vi "PathPlanner_Path_ToPathFile.vi"(9 "FileName":string="path1.path", 11 "PathPlannerPath":T7={"Reversed"=FALSE, "RotationTargets"=[], "ConstraintZones"=[], "EventMarkers"=[], "GlobalConstraints"={"MaxVelocityMps;"=0.0, "MaxAccelerationMpsSq;"=0.0, "MaxAngularVelRadPsEc;"=0.0, "MaxAngularAccRadPSecSq"=0.0, "Exists"=FALSE, "Unlimited"=FALSE, "NominalVoltageVolts"=12.0}, "GoalEndState"={"VelocityMPS"=0.0, "Rotation"={"VALUE"=0.0, "COS"=1.0, "SIN"=0.0}}, "AllPoints"=[], "Name"="", "Waypoints"=[], "PointTowardsZones"=[], "IdealStartingState"={"VelocityMPS"=0.0, "Rotation"={"VALUE"=1.0, "COS"=0.0, "SIN"=0.0}}, "IsChoreoPath"=FALSE, "PreventFlipping"=FALSE} {"IdealStartingState"."Rotation"."SIN" format="%13.4f"; "IdealStartingState"."Rotation"."COS" format="%13.4f"; "IdealStartingState"."Rotation"."VALUE" format="%13.4f"; "PointTowardsZones"."TargetPosition"."Y" format="%14.3f"; "PointTowardsZones"."TargetPosition"."X" format="%14.3f"; "PointTowardsZones"."RotationOffset"."SIN" format="%13.4f"; "PointTowardsZones"."RotationOffset"."COS" format="%13.4f"; "PointTowardsZones"."RotationOffset"."VALUE" format="%13.4f"; "Waypoints"."nextControl"."Y" format="%14.3f"; "Waypoints"."nextControl"."X" format="%14.3f"; "Waypoints"."anchor"."Y" format="%14.3f"; "Waypoints"."anchor"."X" format="%14.3f"; "Waypoints"."prevControl"."Y" format="%14.3f"; "Waypoints"."prevControl"."X" format="%14.3f"; "AllPoints"."RotationTarget"."rotation"."SIN" format="%13.4f"; "AllPoints"."RotationTarget"."rotation"."COS" format="%13.4f"; "AllPoints"."RotationTarget"."rotation"."VALUE" format="%13.4f"; "AllPoints"."Position"."Y" format="%14.3f"; "AllPoints"."Position"."X" format="%14.3f"; "GoalEndState"."Rotation"."SIN" format="%13.4f"; "GoalEndState"."Rotation"."COS" format="%13.4f"; "GoalEndState"."Rotation"."VALUE" format="%13.4f"; "RotationTargets"."rotation"."SIN" format="%13.4f"; "RotationTargets"."rotation"."COS" format="%13.4f"; "RotationTargets"."rotation"."VALUE" format="%13.4f"}) -> (0 "error out":errorcluster, 4 "Full Filename":string)   [LabVIEW 2019, in "PathPlanner24.lvlib"]
doc: "Write a path to a path file in storage. The path normally has a .PATH extension. Internally this file is formatted as JSON.\n\nInputs: \n - Path - cluster - PathPlannerPath created from the given file name\n - filename - string - The name of the path to write. Existing files will be overwritten.\n\nOutputs:\n - Error out - cluster - Error cluster\n - Full Filename - string - fully qualified file name.\n\nNotes on file naming:\n - The file name must include the extention. \".csv\" is not automatically appended to the name. \n - The file name can be a simple file or an absolute path. If a simple file name is used the default path on the RoboRIO is: \"home:\\lvuser\\natinst\\LabVIEW Data\". On a Windows PC the default path is the LabVIEW default directory. Normally this is: “%HOMEDRIVE%%HOMEPATH%\\Documents\\LabView Data\".\n - Filenames on the RoboRIO, which runs Linux, are case sensitive."
uses:
  PathPlanner24.lvlib
  TypeDef/PathPlannerPath.ctl
  TypeDef/PathPlannerRotationTarget.ctl
  <vilib>/Rock Robotics/WPI/ThirdParty/JAS_Junk/TrajLib/TypeDef/ROTATION2D.ctl
  TypeDef/PathPlannerConstraintsZone.ctl
  TypeDef/PathPlannerPathConstraints.ctl
  TypeDef/PathPlannerEventMarker.ctl
  TypeDef/PathPlannerCommandUtil.ctl
  ENum/PathPlanner_CommandUtil_Type_ENUM.ctl
  TypeDef/PathPlannerGoalEndState.ctl
  TypeDef/PathPlannerPathPoint.ctl
  <vilib>/Rock Robotics/WPI/ThirdParty/JAS_Junk/TrajLib/TypeDef/TRANSLATION2D.ctl
  TypeDef/PathPlannerWaypoint.ctl
  TypeDef/PathPlannerPointTowardsZone.ctl
  TypeDef/PathPlannerIdealStartingState.ctl
  <vilib>/Rock Robotics/WPI/ThirdParty/JAS_Junk/TrajLib/Rotation2d_GetRadians.vi
  <vilib>/Rock Robotics/WPI/ThirdParty/JAS_Junk/TrajLib/Conv_Radians_Deg.vi
  <vilib>/Rock Robotics/WPI/ThirdParty/JAS_Junk/TrajLib/Trajectory_Library.lvlib
panel:
  in  "?":T1={"name"="", "waypointRelativePos"=0.0, "command"={"type"="", "data"={"commands"=[]}}, "endWaypointRelativePos"=-1.0}
  in  "constraintZones 2":T2
  in  "waypoint":T3={"anchor"={"x"=1e+30, "y"=1e+31}, "prevControl"={"x"=1e+30, "y"=1e+31}, "nextControl"={"x"=1e+30, "y"=1e+31}, "isLocked"=FALSE}
  out "JSON string":string
  in  "constraintZones":T4
  in  "?":T5
  in  "?":T6={"version"="2025.0", "reversed"=FALSE, "globalConstraints"={"maxVelocity"=1.0, "maxAcceleration"=1.0, "maxAngularVelocity"=1.0, "maxAngularAcceleration"=1.0, "nominalVoltage"=1.0, "unlimited"=FALSE}, "goalEndState"={"velocity"=1.0, "rotation"=1.0}, "waypoints"=[], "constraintZones"=[], "rotationTargets"=[], "idealStartingState"={"velocity"=0.0, "rotation"=0.0}, "pointTowardsZones"=[], "useDefaultConstraints"=FALSE, "eventMarkers"=[]}
  in  "error in (no error)":errorcluster
  # "Constraint Zones"
  # "PointTowardsZones"
  # "Rotation Targets"
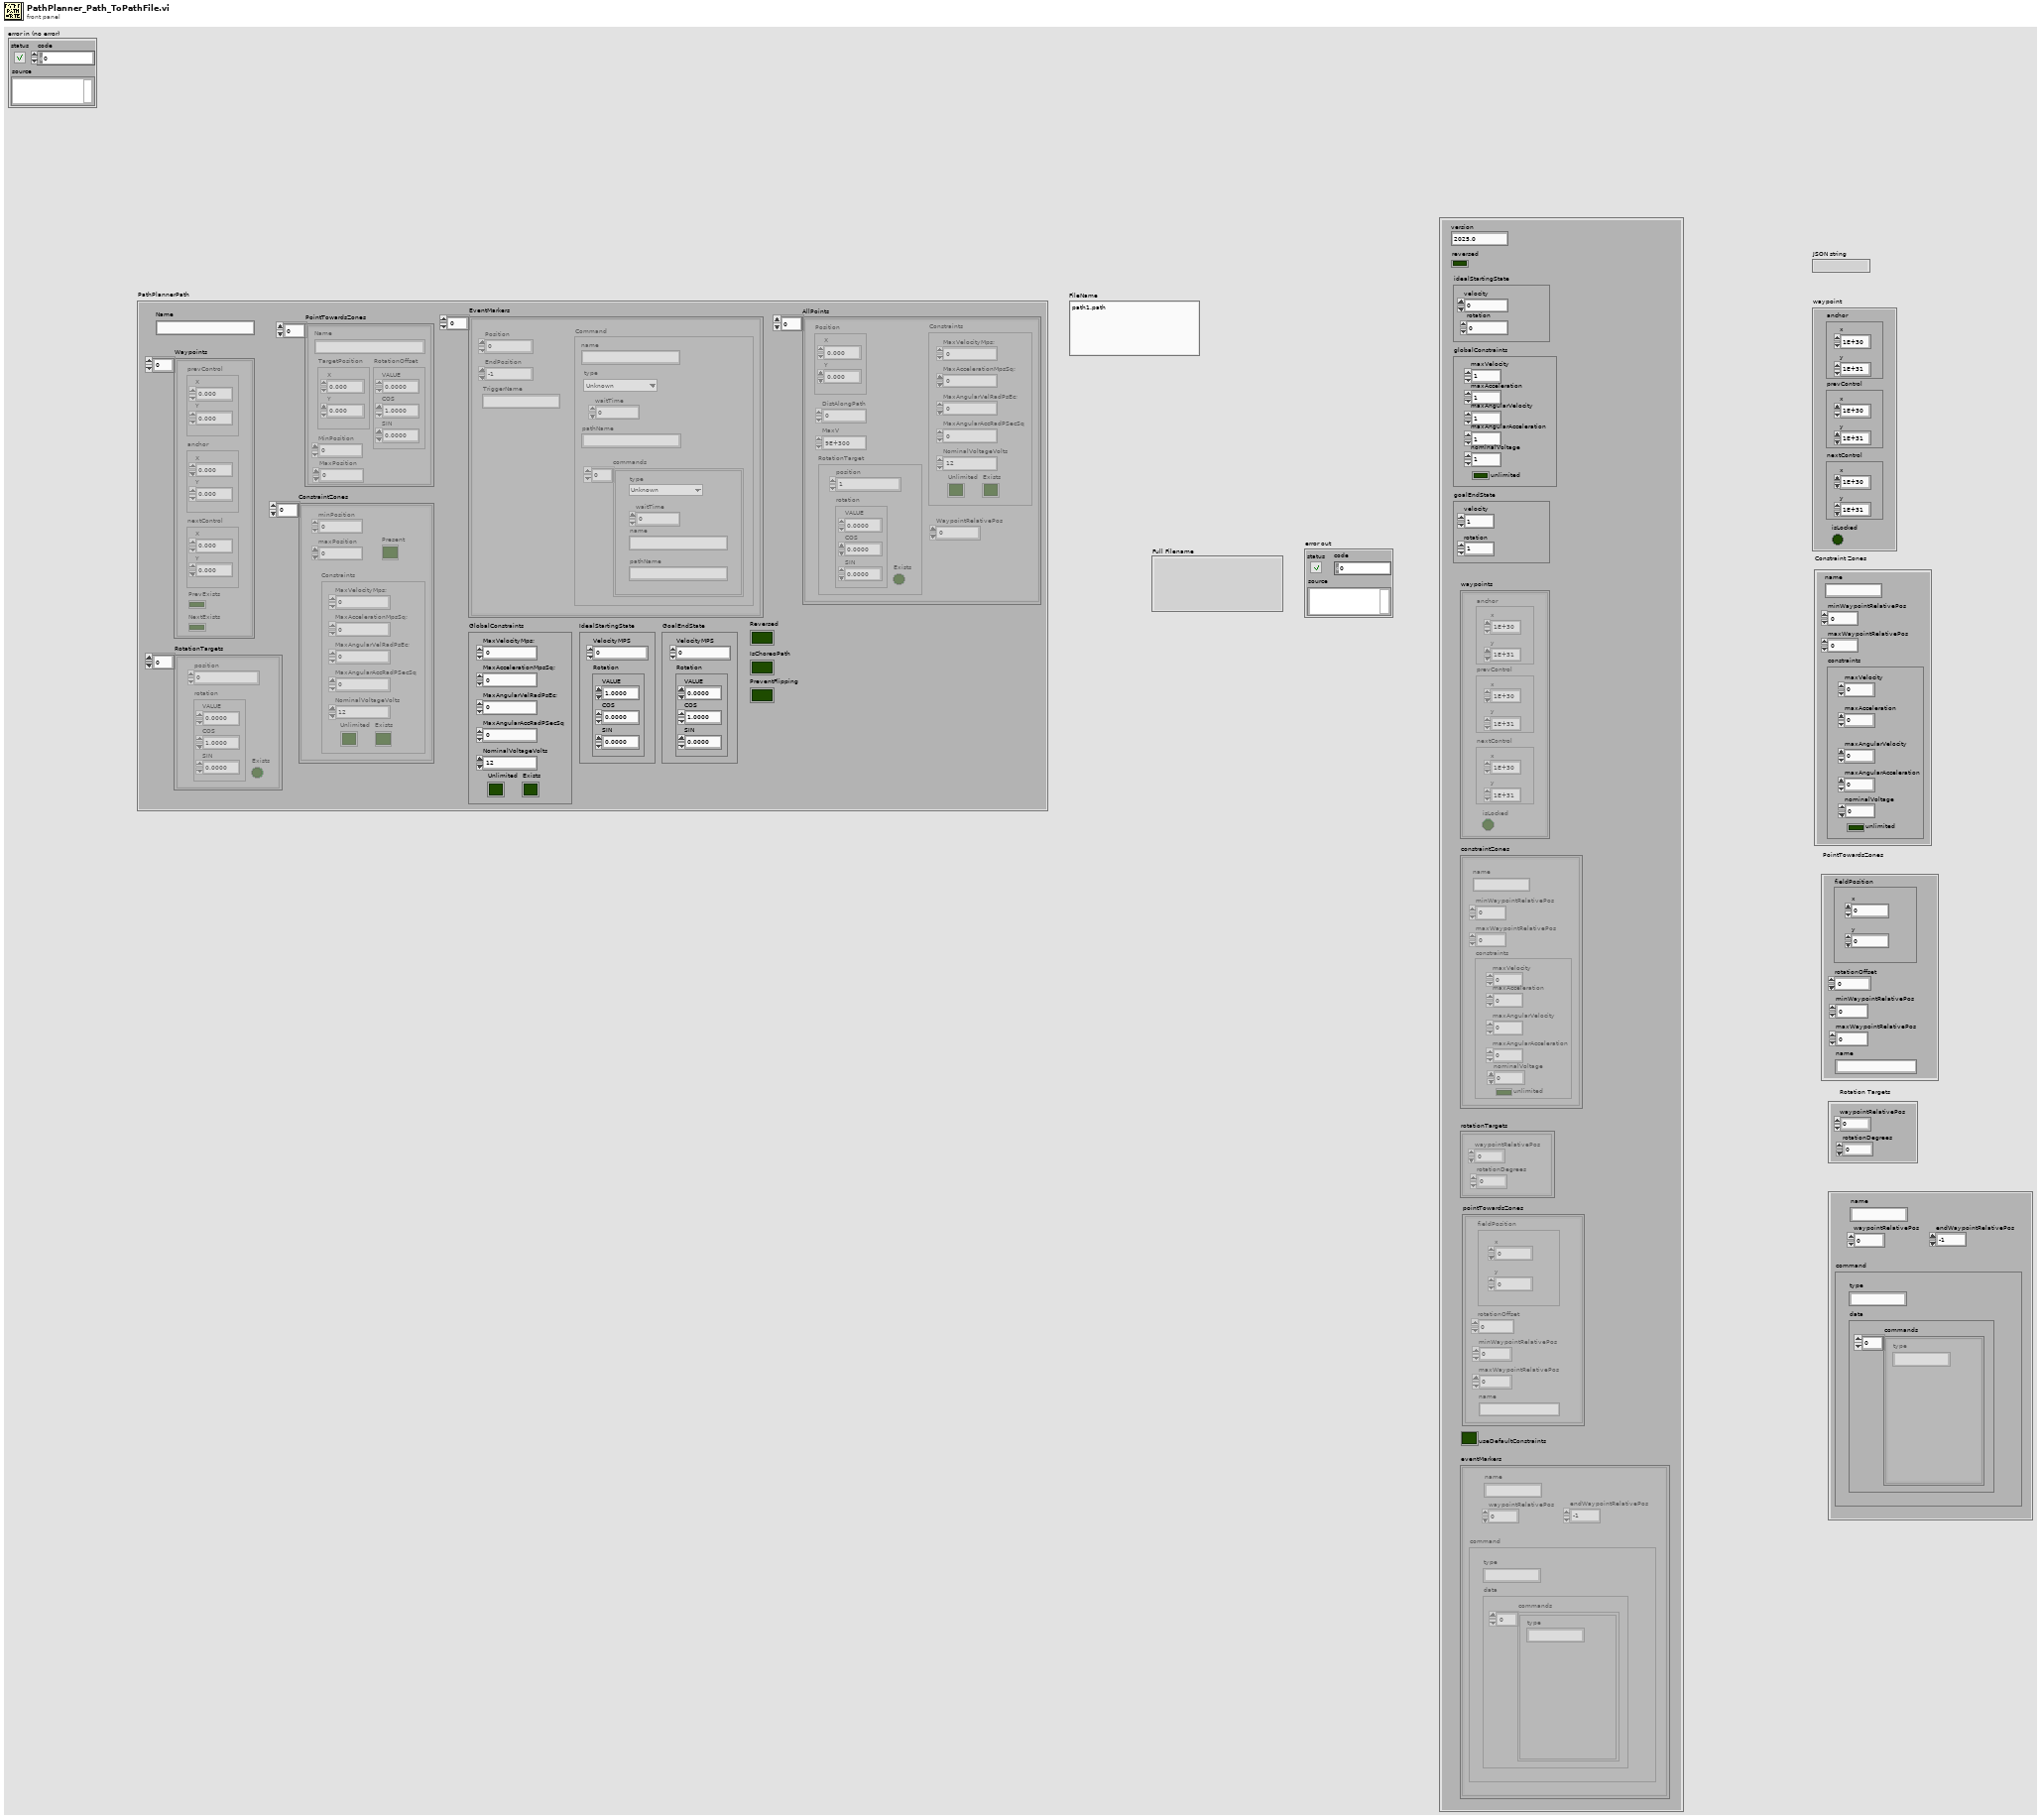
[diagram p1: front panel]
types:
  T1 = cluster{"name":string, "waypointRelativePos":dbl, "command":cluster{"type":string, "data":cluster{"commands":cluster{"type":string}[]}}, "endWaypointRelativePos":dbl}
  T2 = cluster{"fieldPosition":cluster{"x":dbl, "y":dbl}, "rotationOffset":dbl, "minWaypointRelativePos":dbl, "maxWaypointRelativePos":dbl, "name":string}
  T3 = cluster{"anchor":cluster{"x":dbl, "y":dbl}, "prevControl":cluster{"x":dbl, "y":dbl}, "nextControl":cluster{"x":dbl, "y":dbl}, "isLocked":bool}
  T4 = cluster{"name":string, "minWaypointRelativePos":dbl, "maxWaypointRelativePos":dbl, "constraints":cluster{"maxVelocity":dbl, "maxAcceleration":dbl, "maxAngularVelocity":dbl, "maxAngularAcceleration":dbl, "nominalVoltage":dbl, "unlimited":bool}}
  T5 = cluster{"waypointRelativePos":dbl, "rotationDegrees":dbl}
  T6 = cluster{"version":string, "reversed":bool, "globalConstraints":cluster{"maxVelocity":dbl, "maxAcceleration":dbl, "maxAngularVelocity":dbl, "maxAngularAcceleration":dbl, "nominalVoltage":dbl, "unlimited":bool}, "goalEndState":cluster{"velocity":dbl, "rotation":dbl}, "waypoints":cluster{"anchor":cluster{"x":dbl, "y":dbl}, "prevControl":cluster{"x":dbl, "y":dbl}, "nextControl":cluster{"x":dbl, "y":dbl}, "isLocked":bool}[], "constraintZones":cluster{"name":string, "minWaypointRelativePos":dbl, "maxWaypointRelativePos":dbl, "constraints":cluster{"maxVelocity":dbl, "maxAcceleration":dbl, "maxAngularVelocity":dbl, "maxAngularAcceleration":dbl, "nominalVoltage":dbl, "unlimited":bool}}[], "rotationTargets":cluster{"waypointRelativePos":dbl, "rotationDegrees":dbl}[], "idealStartingState":cluster{"velocity":dbl, "rotation":dbl}, "pointTowardsZones":cluster{"fieldPosition":cluster{"x":dbl, "y":dbl}, "rotationOffset":dbl, "minWaypointRelativePos":dbl, "maxWaypointRelativePos":dbl, "name":string}[], "useDefaultConstraints":bool, "eventMarkers":cluster{"name":string, "waypointRelativePos":dbl, "command":cluster{"type":string, "data":cluster{"commands":cluster{"type":string}[]}}, "endWaypointRelativePos":dbl}[]}
  T7 = typedef "PathPlanner24.lvlib/PathPlannerPath.ctl" = cluster{"Reversed":bool, "RotationTargets":T8[], "ConstraintZones":T10[], "EventMarkers":T12[], "GlobalConstraints":T11, "GoalEndState":T15, "AllPoints":T16[], "Name":string, "Waypoints":T18[], "PointTowardsZones":T19[], "IdealStartingState":T20, "IsChoreoPath":bool, "PreventFlipping":bool}
  T8 = typedef "PathPlanner24.lvlib/PathPlannerRotationTarget.ctl" = cluster{"position":dbl, "rotation":T9, "Exists":bool}
  T9 = typedef "Trajectory_Library.lvlib/ROTATION2D.ctl" = cluster{"VALUE":dbl, "COS":dbl, "SIN":dbl}
  T10 = typedef "PathPlanner24.lvlib/PathPlannerConstraintsZone.ctl" = cluster{"minPosition":dbl, "maxPosition":dbl, "Constraints":T11, "Present":bool}
  T11 = typedef "PathPlanner24.lvlib/PathPlannerPathConstraints.ctl" = cluster{"MaxVelocityMps;":dbl, "MaxAccelerationMpsSq;":dbl, "MaxAngularVelRadPsEc;":dbl, "MaxAngularAccRadPSecSq":dbl, "Exists":bool, "Unlimited":bool, "NominalVoltageVolts":dbl}
  T12 = typedef "PathPlanner24.lvlib/PathPlannerEventMarker.ctl" = cluster{"Position":dbl, "Command":T13, "TriggerName":string, "EndPosition":dbl}
  T13 = typedef "PathPlanner24.lvlib/PathPlannerCommandUtil.ctl" = cluster{"waitTime":dbl, "name":string, "pathName":string, "commands":cluster{"type":T14, "waitTime":dbl, "name":string, "pathName":string}[], "type":T14}
  T14 = typedef "PathPlanner24.lvlib/PathPlanner_CommandUtil_Type_ENUM.ctl" = enum16{"Unknown", "Wait", "Named", "Path", "Sequential", "Parallel", "Race", "Deadline", "PointTowardsZoneEnter", "PointTowardsZoneExit", "TriggerEventStart", "TriggerEventStop", "TriggerEventOneshot"}
  T15 = typedef "PathPlanner24.lvlib/PathPlannerGoalEndState.ctl" = cluster{"VelocityMPS":dbl, "Rotation":T9}
  T16 = typedef "PathPlanner24.lvlib/PathPlannerPathPoint.ctl" = cluster{"Position":T17, "DistAlongPath":dbl, "MaxV":dbl, "Constraints":T11, "RotationTarget":T8, "WaypointRelativePos":dbl}
  T17 = typedef "Trajectory_Library.lvlib/TRANSLATION2D.ctl" = cluster{"X":dbl, "Y":dbl}
  T18 = typedef "PathPlanner24.lvlib/PathPlannerWaypoint.ctl" = cluster{"prevControl":T17, "anchor":T17, "nextControl":T17, "PrevExists":bool, "NextExists":bool}
  T19 = typedef "PathPlanner24.lvlib/PathPlannerPointTowardsZone.ctl" = cluster{"RotationOffset":T9, "Name":string, "TargetPosition":T17, "MinPosition":dbl, "MaxPosition":dbl}
  T20 = typedef "PathPlanner24.lvlib/PathPlannerIdealStartingState.ctl" = cluster{"VelocityMPS":dbl, "Rotation":T9}
  T21 = cluster{"name":string, "waypointRelativePos":dbl, "command":cluster{"type":string, "data":cluster{"commands":cluster{"type":string}[]}}, "endWaypointRelativePos":dbl}[]
  T22 = cluster{"name":string, "minWaypointRelativePos":dbl, "maxWaypointRelativePos":dbl, "constraints":cluster{"maxVelocity":dbl, "maxAcceleration":dbl, "maxAngularVelocity":dbl, "maxAngularAcceleration":dbl, "nominalVoltage":dbl, "unlimited":bool}}[]
  T23 = cluster{"waypointRelativePos":dbl, "rotationDegrees":dbl}[]
  T24 = cluster{"fieldPosition":cluster{"x":dbl, "y":dbl}, "rotationOffset":dbl, "minWaypointRelativePos":dbl, "maxWaypointRelativePos":dbl, "name":string}[]
  T25 = cluster{"anchor":cluster{"x":dbl, "y":dbl}, "prevControl":cluster{"x":dbl, "y":dbl}, "nextControl":cluster{"x":dbl, "y":dbl}, "isLocked":bool}[]
  T26 = enum16{"open", "replace", "create", "open or create", "replace or create", "replace or create with confirmation"}
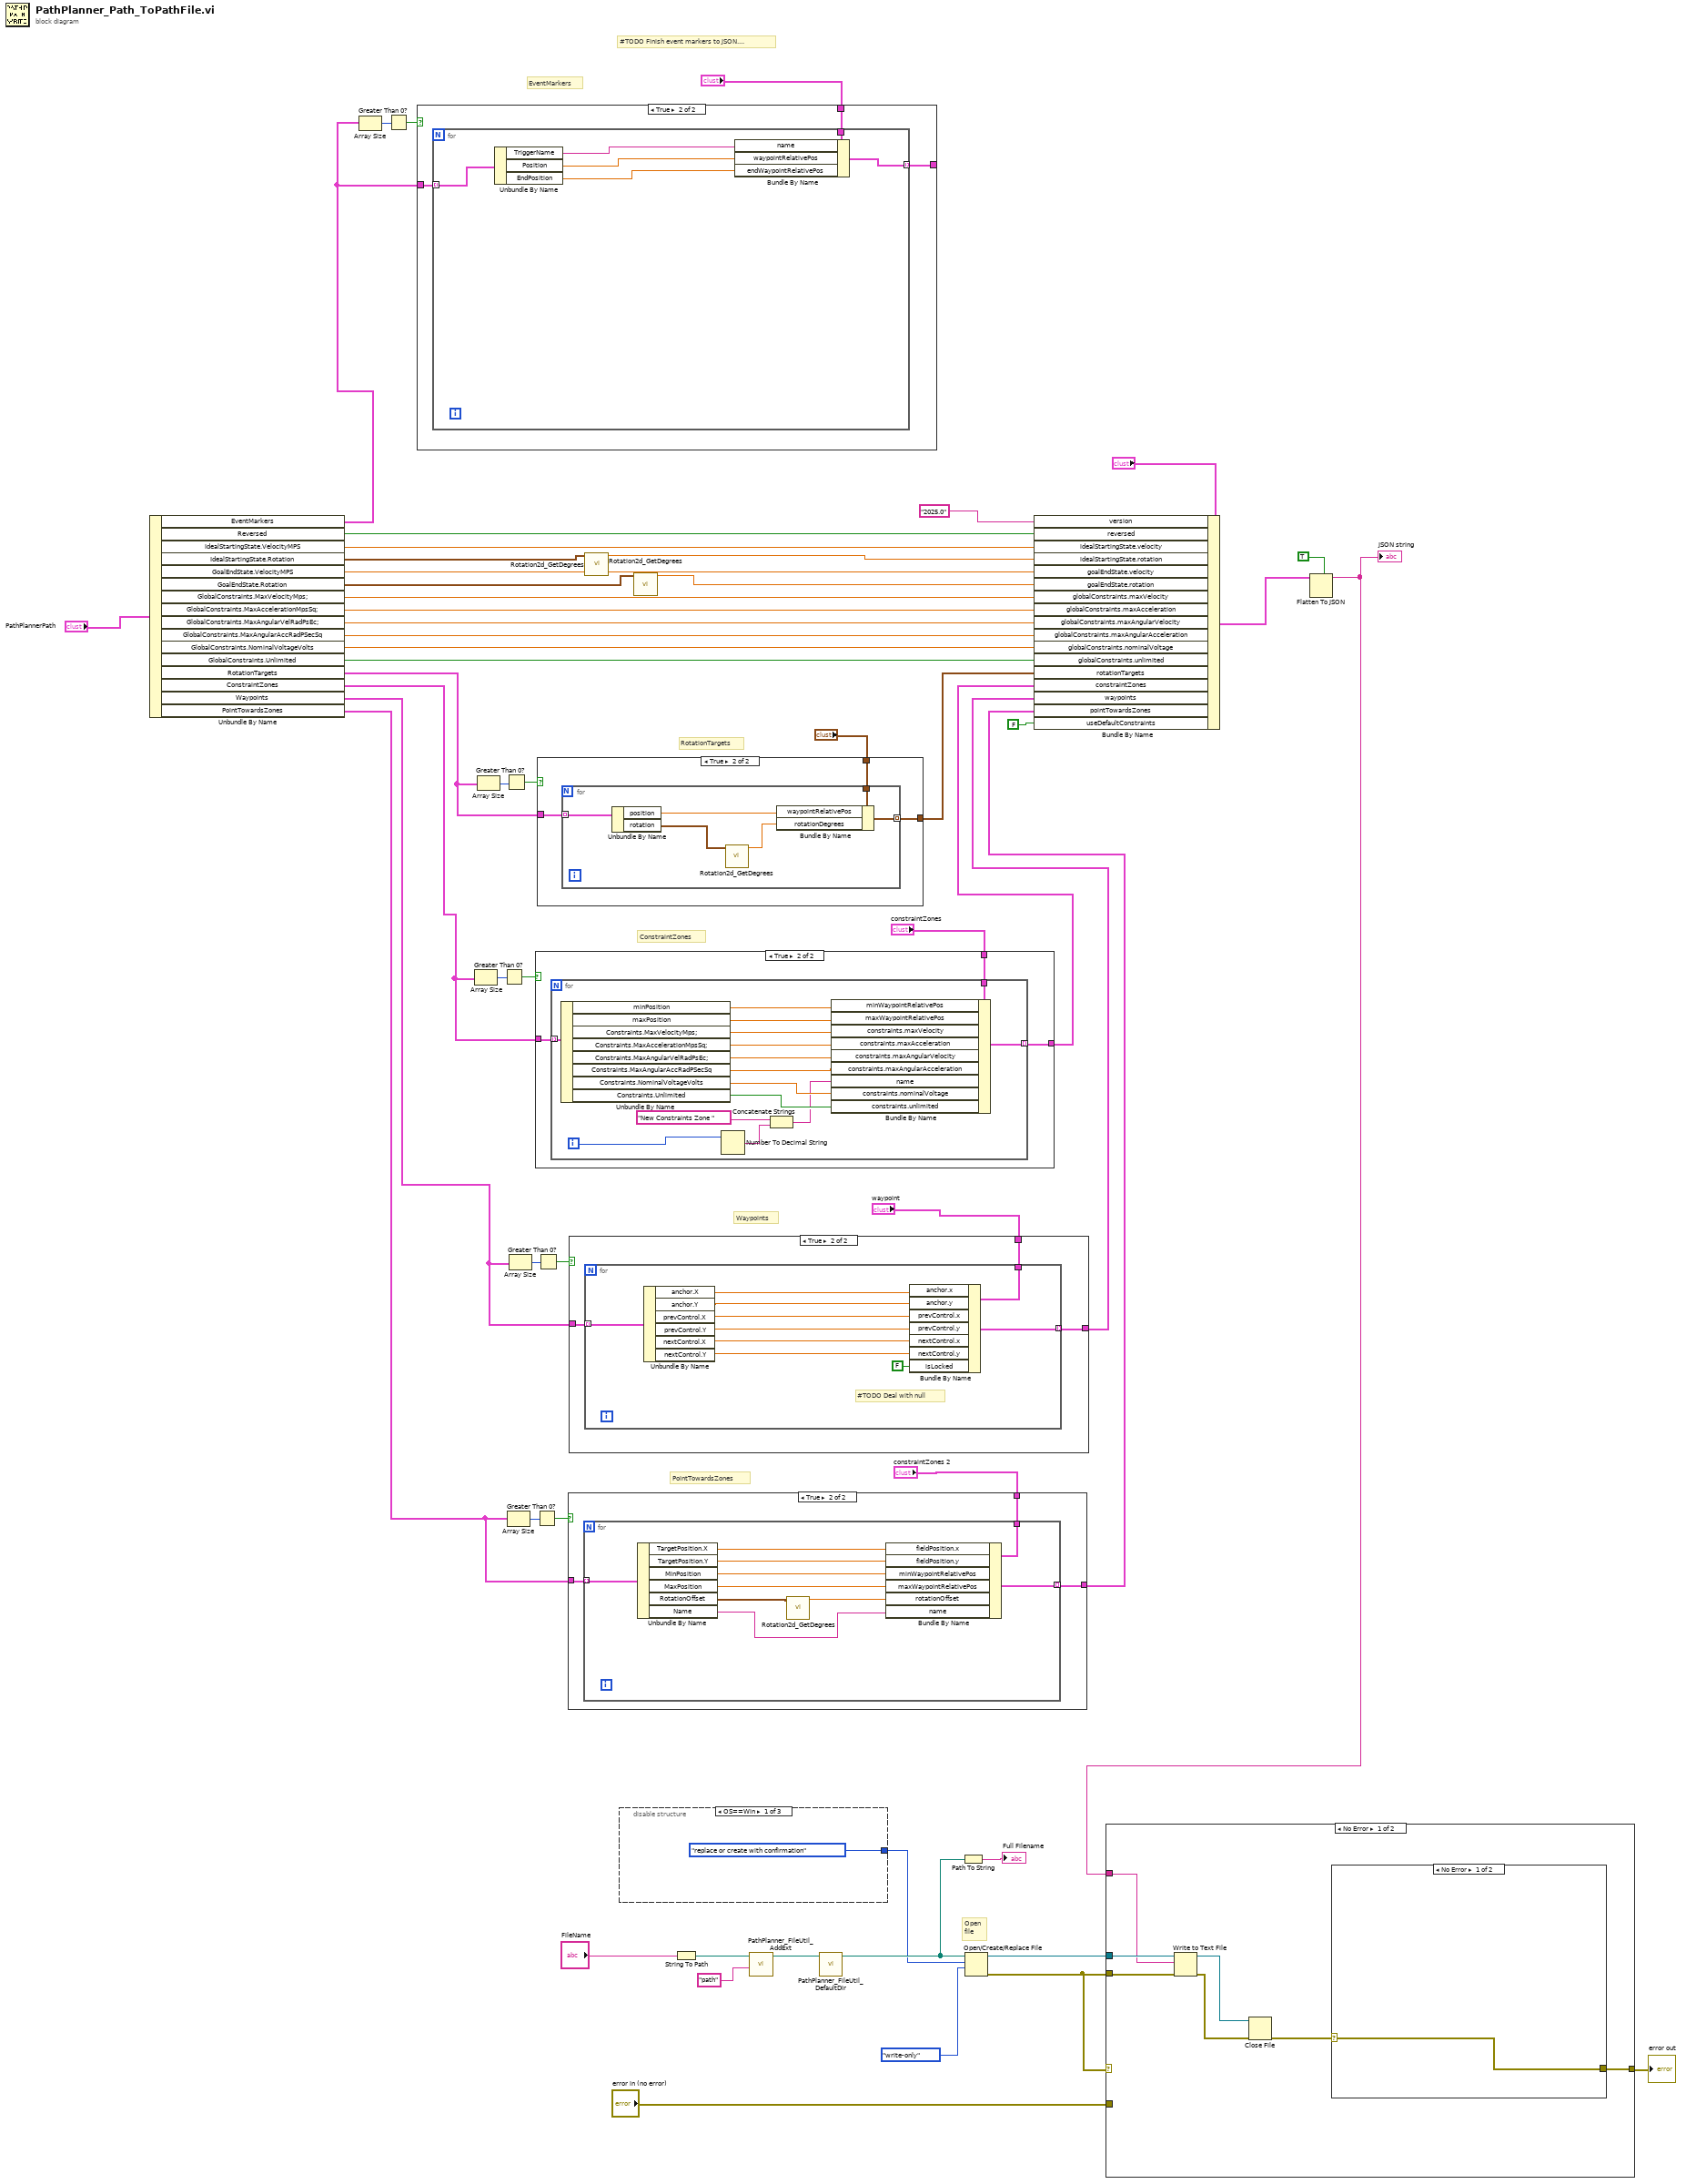
[diagram p0: block diagram]
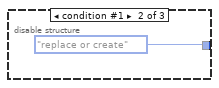
[diagram p2: hidden frame]
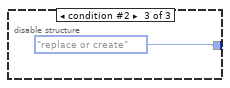
[diagram p3: hidden frame]
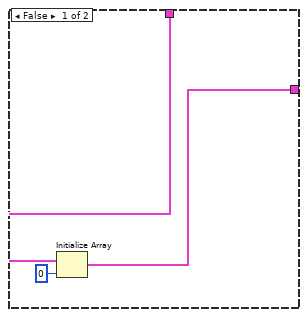
[diagram p4: hidden frame]
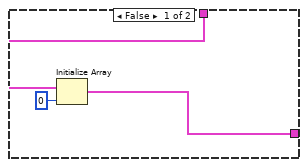
[diagram p5: hidden frame]
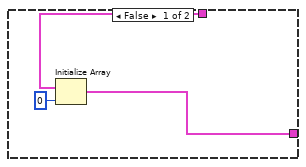
[diagram p6: hidden frame]
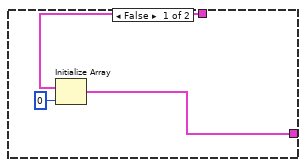
[diagram p7: hidden frame]
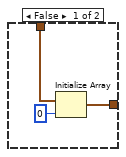
[diagram p8: hidden frame]
diagram:
  # "#TODO Finish event markers to JSON...."
  # "EventMarkers"
  # "PointTowardsZones"
  # "RotationTargets"
  # "Waypoints"
  # "ConstraintZones"
  # "Open\nfile"
  n1 = Unbundle By Name("PathPlannerPath") -> ("EventMarkers"=w6:T12[], "Reversed"=w48:bool, "IdealStartingState.VelocityMPS"=w21:dbl, "IdealStartingState.Rotation"=w23:T9, "GoalEndState.VelocityMPS"=w12:dbl, "GoalEndState.Rotation"=w11:T9, "GlobalConstraints.MaxVelocityMps;"=w47:dbl, "GlobalConstraints.MaxAccelerationMpsSq;"=w46:dbl, "GlobalConstraints.MaxAngularVelRadPsEc;"=w45:dbl, "GlobalConstraints.MaxAngularAccRadPSecSq"=w44:dbl, "GlobalConstraints.NominalVoltageVolts"=w20:dbl, "GlobalConstraints.Unlimited"=w19:bool, "RotationTargets"=w41:T8[], "ConstraintZones"=w34:T10[], "Waypoints"=w27:T18[], "PointTowardsZones"=w15:T19[])
  n2 = Array Size(array=w6) -> (size(s)=w9:i32)
  n3 = Greater Than 0?(x=w9) -> (x > 0?=w8:bool)
  n4 = case shown="True" w8 {
    tunnel: w6 -> [_ w62]
    tunnel: "?" -> [w57 w61]
    tunnel: [w58 w60] -> _
    frame False {
      n5 = Initialize Array(w57, 0 ("dimension size")) -> (w58:T21)
    }
    frame True {
      n6 = for {
        tunnel: w62 -> [w68] mode=indexing
        tunnel: w61 -> [w63]
        tunnel: [w67] -> w60 mode=indexing
        n7 = Unbundle By Name(w68) -> ("TriggerName"=w66:string, "Position"=w65:dbl, "EndPosition"=w64:dbl)
        n8 = Bundle By Name(cluster=w63, "name"=w66, "waypointRelativePos"=w65, "endWaypointRelativePos"=w64) -> (w67:T1)
      }
    }
  }
  n9 = Array Size(array=w34) -> (size(s)=w36:i32)
  n10 = Array Size(array=w41) -> (size(s)=w43:i32)
  n11 = Greater Than 0?(x=w36) -> (x > 0?=w35:bool)
  n12 = Greater Than 0?(x=w43) -> (x > 0?=w42:bool)
  n13 = Array Size(array=w15) -> (size(s)=w18:i32)
  n14 = Array Size(array=w27) -> (size(s)=w29:i32)
  n15 = case shown="True" w35 {
    tunnel: w34 -> [_ w74]
    tunnel: "constraintZones" -> [w71 w73]
    tunnel: [w69 w72] -> w32
    frame False {
      n16 = Initialize Array(w71, 0 ("dimension size")) -> (w69:T22)
    }
    frame True {
      n17 = for {
        tunnel: w74 -> [w89] mode=indexing
        tunnel: w73 -> [w88]
        tunnel: [w86] -> w72 mode=indexing
        i -> [w85]
        n18 = Unbundle By Name(w89) -> ("minPosition"=w87:dbl, "maxPosition"=w84:dbl, "Constraints.MaxVelocityMps;"=w83:dbl, "Constraints.MaxAccelerationMpsSq;"=w82:dbl, "Constraints.MaxAngularVelRadPsEc;"=w81:dbl, "Constraints.MaxAngularAccRadPSecSq"=w80:dbl, "Constraints.NominalVoltageVolts"=w79:dbl, "Constraints.Unlimited"=w78:bool)
        n19 = Number To Decimal String(number=w85) -> (decimal integer string=w77:string)  [unwired: 1 in]
        n20 = Concatenate Strings("New Constraints Zone " ("string"), w77) -> (w76:string)
        n21 = Bundle By Name(cluster=w88, "minWaypointRelativePos"=w87, "maxWaypointRelativePos"=w84, "constraints.maxVelocity"=w83, "constraints.maxAcceleration"=w82, "constraints.maxAngularVelocity"=w81, "constraints.maxAngularAcceleration"=w80, "name"=w76, "constraints.nominalVoltage"=w79, "constraints.unlimited"=w78) -> (w86:T4)
      }
    }
  }
  n22 = Greater Than 0?(x=w18) -> (x > 0?=w17:bool)
  n23 = Greater Than 0?(x=w29) -> (x > 0?=w28:bool)
  n24 = case shown="True" w42 {
    tunnel: w41 -> [_ w95]
    tunnel: "?" -> [w92 w94]
    tunnel: [w90 w93] -> w39
    frame False {
      n25 = Initialize Array(w92, 0 ("dimension size")) -> (w90:T23)
    }
    frame True {
      n26 = for {
        tunnel: w95 -> [w101] mode=indexing
        tunnel: w94 -> [w100]
        tunnel: [w96] -> w93 mode=indexing
        n27 = Unbundle By Name(w101) -> ("position"=w97:dbl, "rotation"=w99:T9)
        n28 = call <vilib>:"Rotation2d_GetDegrees.vi"("in ROTATION"=w99) -> ("AngleDegrees"=w98:dbl)  [unwired: 10 in]
        n29 = Bundle By Name(cluster=w100, "waypointRelativePos"=w97, "rotationDegrees"=w98) -> (w96:T5)
      }
    }
  }
  n30 = case shown="True" w17 {
    tunnel: w15 -> [_ w107]
    tunnel: "constraintZones 2" -> [w102 w106]
    tunnel: [w103 w105] -> w14
    frame False {
      n31 = Initialize Array(w102, 0 ("dimension size")) -> (w103:T24)
    }
    frame True {
      n32 = for {
        tunnel: w107 -> [w117] mode=indexing
        tunnel: w106 -> [w116]
        tunnel: [w115] -> w105 mode=indexing
        n33 = Unbundle By Name(w117) -> ("TargetPosition.X"=w114:dbl, "TargetPosition.Y"=w113:dbl, "MinPosition"=w112:dbl, "MaxPosition"=w111:dbl, "RotationOffset"=w110:T9, "Name"=w108:string)
        n34 = call <vilib>:"Rotation2d_GetDegrees.vi"("in ROTATION"=w110) -> ("AngleDegrees"=w109:dbl)  [unwired: 10 in]
        n35 = Bundle By Name(cluster=w116, "fieldPosition.x"=w114, "fieldPosition.y"=w113, "minWaypointRelativePos"=w112, "maxWaypointRelativePos"=w111, "rotationOffset"=w109, "name"=w108) -> (w115:T2)
      }
    }
  }
  n36 = case shown="True" w28 {
    tunnel: w27 -> [_ w123]
    tunnel: "waypoint" -> [w120 w122]
    tunnel: [w118 w121] -> w25
    frame False {
      n37 = Initialize Array(w120, 0 ("dimension size")) -> (w118:T25)
    }
    frame True {
      n38 = for {
        tunnel: w123 -> [w133] mode=indexing
        tunnel: w122 -> [w132]
        tunnel: [w131] -> w121 mode=indexing
        # "#TODO Deal with null"
        n39 = Unbundle By Name(w133) -> ("anchor.X"=w130:dbl, "anchor.Y"=w129:dbl, "prevControl.X"=w128:dbl, "prevControl.Y"=w127:dbl, "nextControl.X"=w126:dbl, "nextControl.Y"=w125:dbl)
        n40 = Bundle By Name(cluster=w132, "anchor.x"=w130, "anchor.y"=w129, "prevControl.x"=w128, "prevControl.y"=w127, "nextControl.x"=w126, "nextControl.y"=w125, "isLocked"=FALSE) -> (w131:T3)
      }
    }
  }
  n41 = call <vilib>:"Rotation2d_GetDegrees.vi"("in ROTATION"=w23) -> ("AngleDegrees"=w22:dbl)  [unwired: 10 in]
  n42 = disable-structure shown="OS==Win" {
    disable-tunnel: [T26."replace or create with confirmation" ("operation (0:open)") T26."replace or create" ("operation (0:open)") T26."replace or create" ("operation (0:open)")] -> w1
    frame condition #0 (active) {
    }
    frame condition #1 {
    }
    frame condition #2 {
    }
  }
  n43 = call <vilib>:"Rotation2d_GetDegrees.vi"("in ROTATION"=w11) -> ("AngleDegrees"=w10:dbl)  [unwired: 10 in]
  n44 = String To Path(string="FileName") -> (path=w5:path)
  n45 = call "PathPlanner_FileUtil_AddExt.vi"("Extension"="path", "Path in"=w5) -> ("Path out"=w4:path)  [unwired: 9 in]
  n46 = call "PathPlanner_FileUtil_DefaultDir.vi"("Path in"=w4) -> ("Path Out"=w3:path)  [unwired: 10 in]
  n47 = Path To String(path=w3) -> (string=→"Full Filename":string)
  n48 = Open/Create/Replace File(file path (use dialog)=w3, operation (0:open)=w1, access (0:read/write)=enum16{"read/write", "read-only", "write-only"}."write-only") -> (refnum out=w54:refnum<file>, error out=w30:errorcluster)  [unwired: 3 in, 1 out]
  n49 = Bundle By Name(cluster="?", "version"="2025.0", "reversed"=w48, "idealStartingState.velocity"=w21, "idealStartingState.rotation"=w22, "goalEndState.velocity"=w12, "goalEndState.rotation"=w10, "globalConstraints.maxVelocity"=w47, "globalConstraints.maxAcceleration"=w46, "globalConstraints.maxAngularVelocity"=w45, "globalConstraints.maxAngularAcceleration"=w44, "globalConstraints.nominalVoltage"=w20, "globalConstraints.unlimited"=w19, "rotationTargets"=w39, "constraintZones"=w32, "waypoints"=w25, "pointTowardsZones"=w14, "useDefaultConstraints"=FALSE) -> (w37:T6)
  n50 = Flatten To JSON(enable LabVIEW extensions? (T)=TRUE, anything=w37) -> (JSON string=w31:string)  [unwired: 1 in, 1 out]
  "JSON string" <- w31
  n51 = case shown="No Error" w30 {
    selector: w30 -> [_ w146]
    tunnel: w54 -> [w141 _]
    tunnel: [w142 w146] -> w51
    tunnel: "error in (no error)" -> [_ _]
    tunnel: w31 -> [w140 _]
    tunnel: w30 -> [w139 _]
    frame No Error {
      n52 = Write to Text File(file (use dialog)=w141, text=w140, error in=w139) -> (refnum out=w137:refnum<file>, error out=w138:errorcluster)  [unwired: 1 in, 1 out]
      n53 = Close File(refnum=w137, error in=w138) -> (error out=w143:errorcluster)  [unwired: 1 out]
      n54 = case shown="No Error" w143 {
        selector: w143 -> [w144 w145]
        tunnel: [w144 w145] -> w142
        frame No Error {
        }
        frame Error {
        }
      }
    }
    frame Error {
    }
  }
  "error out" <- w51
